vi "Interface.vi"() -> ()   [LabVIEW 2016, in "Socket Auto Connect.lvclass"]
uses:
  Socket Auto Connect.lvclass
  Robot/Universal Robot/Universal Robot.lvclass
  C:/_Code/Development/URLabVIEWInterface/Classes/Application/Application Interfaces/Application Interface/Application Interface.lvclass
  Socket Auto Connect.lvclass/Socket Auto Connect.ctl
  Client Interfaces/Socket Communication/Socket Communication.lvclass
  Application.lvclass
  Application Interface/Application Interface.lvclass
panel:
  out "connected":bool
  out "running":bool
  out "Data Viewer":string
  in  "interface":refnum<class "Socket Auto Connect.lvclass">
  in  "robot":refnum<class "Universal Robot.lvclass">
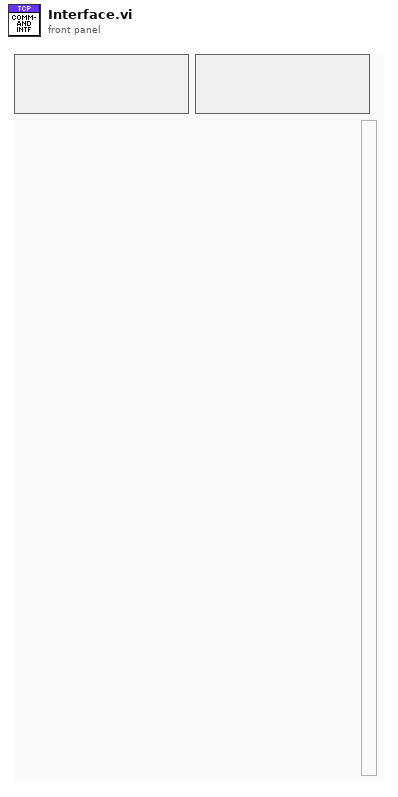
[diagram p1: front panel]
types:
  T1 = typedef "Application.lvclass/FrontPanelControls.ctl" = cluster{"Operation Interface":refnum<vi>, "Program Interface":refnum<vi>, "Command Interface":refnum<vi>, "Socket Interface":refnum<vi>}
  T2 = typedef "Universal Robot.lvclass/ProgramStatus.ctl" = cluster{"Loaded Program":string, "Valid Program":bool, "Program State":T3, "Running":bool}
  T3 = typedef "Universal Robot.lvclass/ProgramState.ctl" = enum16{"STOPPED", "PLAYING", "PAUSE"}
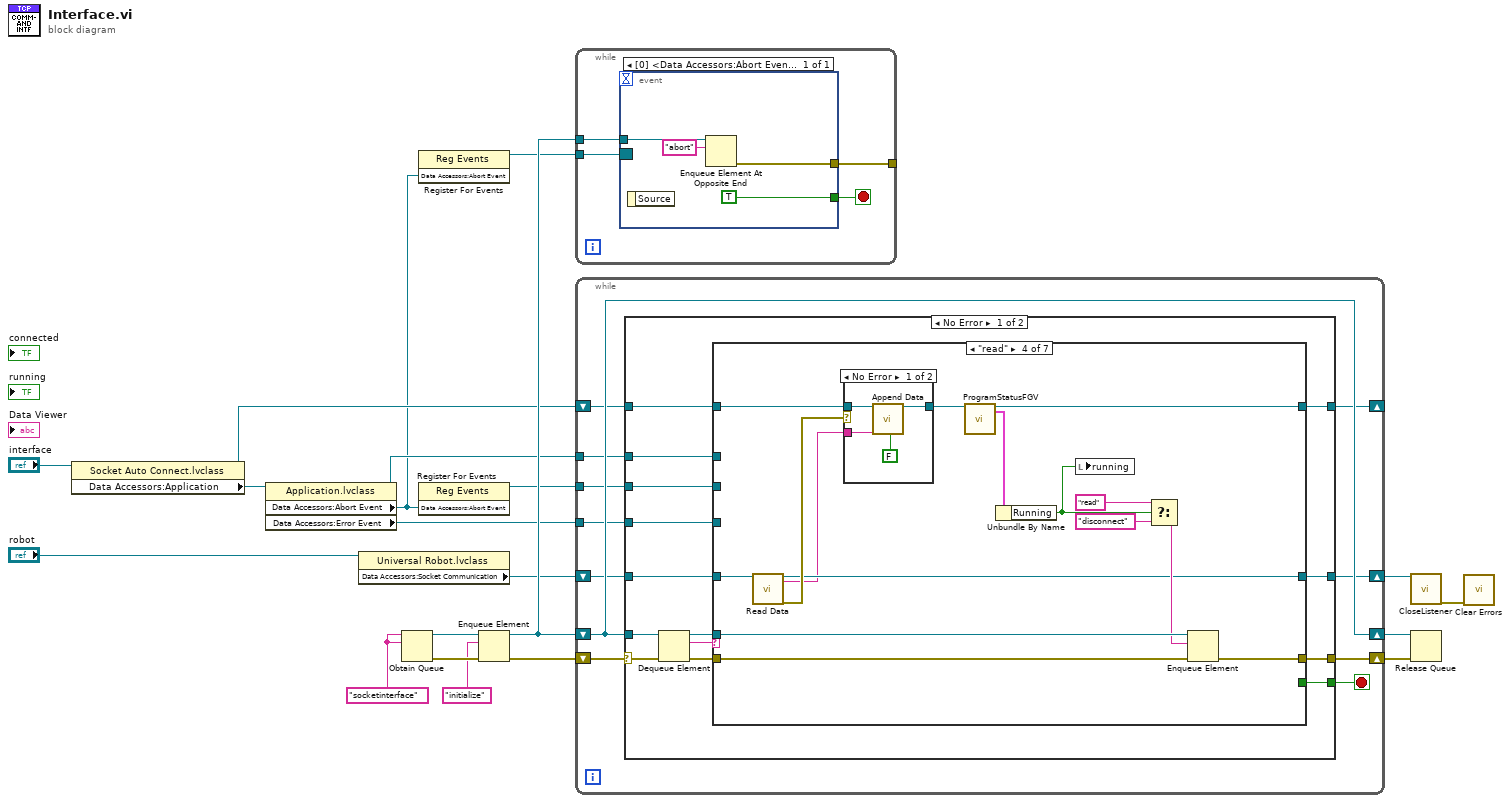
[diagram p0: block diagram]
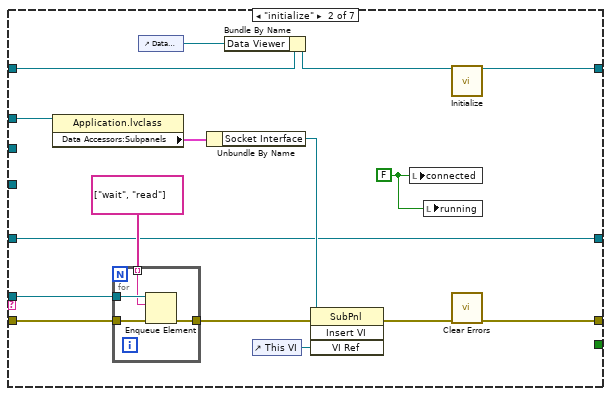
[diagram p3: hidden frame]
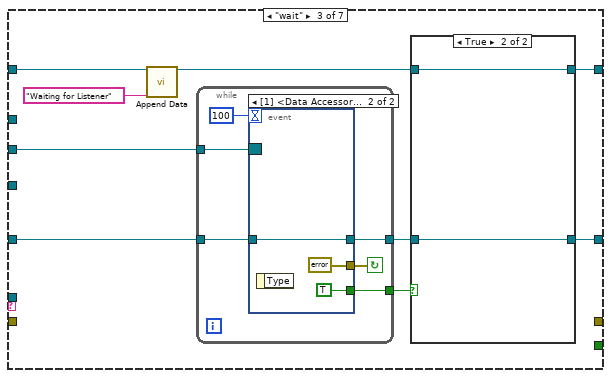
[diagram p4: hidden frame]
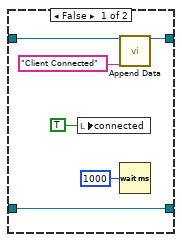
[diagram p5: hidden frame]
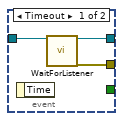
[diagram p6: hidden frame]
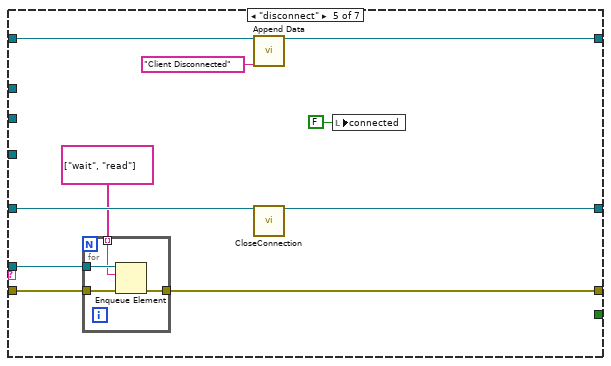
[diagram p8: hidden frame]
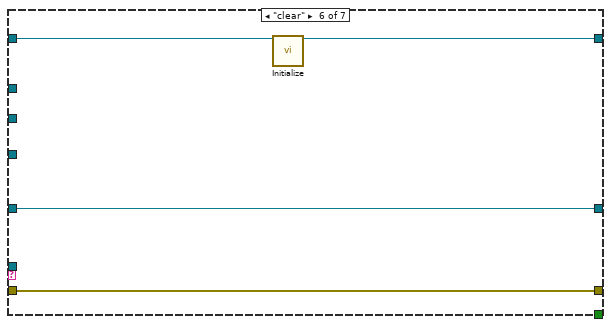
[diagram p9: hidden frame]
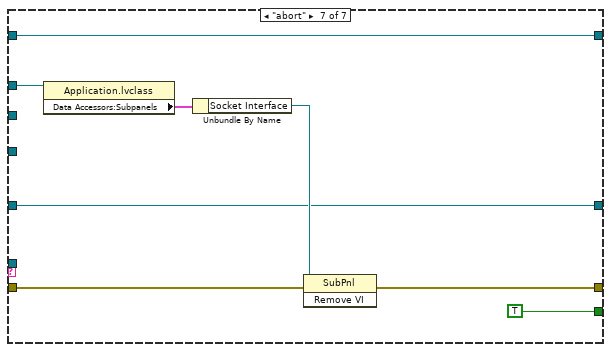
[diagram p10: hidden frame]
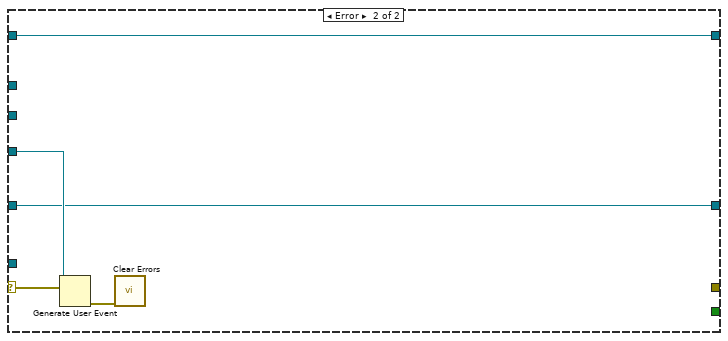
[diagram p11: hidden frame]
diagram:
  w15 = "socketinterface" ("name (unnamed)")
  n1 = property class="Socket Auto Connect.lvclass"(reference="interface") -> (reference out=w9:refnum<class "Socket Auto Connect.lvclass">, "Data Accessors:Application"=w12:refnum<class "Application.lvclass">)  [unwired: 1 in, 1 out]
  n2 = property class="Application.lvclass"(reference=w12) -> (reference out=w8:refnum<class "Application.lvclass">, "Data Accessors:Abort Event"=w3:refnum<user-event>, "Data Accessors:Error Event"=w11:refnum<user-event>)  [unwired: 1 in, 1 out]
  n3 = property class="Universal Robot.lvclass"(reference="robot") -> ("Data Accessors:Socket Communication"=w6:refnum<class "Socket Communication.lvclass">)  [unwired: 1 in, 2 out]
  n4 = Obtain Queue(name (unnamed)=w15, element data type=w15) -> (queue out=w19:refnum<queue>, error out=w20:errorcluster)  [unwired: 3 in, 1 out]
  n5 = register-events(w3) -> (reference out=w4:refnum<event-registration>)  [unwired: 2 in, 1 out]
  n6 = register-events(w3) -> (reference out=w5:refnum<event-registration>)  [unwired: 2 in, 1 out]
  n7 = Enqueue Element(queue=w19, element="initialize", error in (no error)=w20) -> (queue out=w16:refnum<queue>, error out=w17:errorcluster)  [unwired: 1 in, 1 out]
  n8 = while {
    tunnel: w16 -> [w24]
    tunnel: w4 -> [w23]
    tunnel: [w22] -> _
    stop <- w21 stop-if-true
    n9 = event shown="[0] <Data Accessors:Abort Event>: User Event" {
      selector: w23 -> [_]
      dyn-events: _ -> [_]
      timeout: _ -> [_]
      tunnel: w24 -> [w28]
      tunnel: [w27] -> w22
      tunnel: [TRUE] -> w21
      event User Event {
        n10 = event-data() -> ()  [unwired: 1 in, 1 out]
        n11 = Enqueue Element At Opposite End(queue=w28, element="abort") -> (error out=w27:errorcluster)  [unwired: 2 in, 2 out]
      }
    }
  }
  n12 = while {
    shift-right: [w37] -> w13
    shift-left: w17 -> [w39]
    shift-right: [w38] -> w14
    shift-left: w16 -> [w38]
    tunnel: w11 -> [w35]
    tunnel: w5 -> [w34]
    shift-right: [w32] -> _
    shift-left: w9 -> [w33]
    tunnel: w8 -> [w31]
    shift-right: [w29] -> w2
    shift-left: w6 -> [w30]
    stop <- w36 stop-if-true
    n13 = case shown="No Error" w39 {
      selector: w39 -> [w52 w156]
      tunnel: w38 -> [w53 _]
      tunnel: [w48 _] -> w37
      tunnel: [w47 _] -> w36
      tunnel: w35 -> [w46 w154]
      tunnel: w34 -> [w45 _]
      tunnel: w33 -> [w44 w153]
      tunnel: [w43 w153] -> w32
      tunnel: w31 -> [w42 _]
      tunnel: w30 -> [w41 w152]
      tunnel: [w40 w152] -> w29
      frame No Error {
        n14 = Dequeue Element(queue=w53, error in (no error)=w52) -> (queue out=w49:refnum<queue>, element=w50:string, error out=w51:errorcluster)  [unwired: 1 in, 1 out]
        n15 = case shown="\"read\"" w50 {
          tunnel: w51 -> [w56 w63 _ w113 w127 w142 w150]
          tunnel: w49 -> [_ w64 _ w114 w128 _ _]
          tunnel: [w56 w58 _ w111 w126 w142 w149] -> w48
          tunnel: [_ _ _ _ _ _ TRUE] -> w47
          tunnel: w46 -> [_ _ _ _ _ _ _]
          tunnel: w45 -> [_ _ w85 _ _ _ _]
          tunnel: w44 -> [w55 w69 w84 w116 w135 w141 w146]
          tunnel: [w55 w67 w81 w120 w134 w140 w146] -> w43
          tunnel: w42 -> [_ w65 _ _ _ _ w145]
          tunnel: w41 -> [w54 w57 w79 w118 w131 w143 w144]
          tunnel: [w54 w57 w77 w107 w130 w143 w144] -> w40
          frame Default {
          }
          frame "initialize" {
            w60 = FALSE ("connected")
            n16 = property class="Application.lvclass"(reference=w65) -> ("Data Accessors:Subpanels"=w71:T1)  [unwired: 1 in, 2 out]
            n17 = for {
              tunnel: w64 -> [w76]
              tunnel: w63 -> [w75]
              tunnel: [w74] -> w62
              tunnel: string[] ["wait", "read"] -> [w73] mode=indexing
              n18 = Enqueue Element(queue=w76, element=w73, error in (no error)=w75) -> (error out=w74:errorcluster)  [unwired: 1 in, 2 out]
            }
            n19 = control-ref of="Data Viewer"() -> (w68:refnum<vi>)
            n20 = Unbundle By Name(w71) -> ("Socket Interface"=w70:refnum<vi>)
            n21 = Bundle By Name(cluster=w69, "Data Viewer"=w68) -> (w66:refnum<class "Socket Auto Connect.lvclass">)
            n22 = control-ref of="This VI"() -> (w72:refnum<vi>)
            n23 = invoke class="SubPnl" method="Insert VI"(reference=w70, error in=w62, "VI Ref"=w72) -> (error out=w59:errorcluster)  [unwired: 1 in, 3 out]
            n24 = local write "connected"(w60) -> ()
            n25 = local write "running"(w60) -> ()
            n26 = call "Initialize.vi"("Socket Auto Connect in"=w66) -> ("Socket Auto Connect out"=w67:refnum<class "Socket Auto Connect.lvclass">)  [unwired: 17 in, 1 out]
            n27 = call <vilib>:"Clear Errors.vi"("error in (no error)"=w59) -> ("error out"=w58:errorcluster)  [unwired: 5 in, 1 out]
          }
          frame "wait" {
            n28 = call "Append Data.vi"("Socket Auto Connect in"=w84, "String to Append"="Waiting for Listener") -> ("Socket Auto Connect out"=w82:refnum<class "Socket Auto Connect.lvclass">)  [unwired: 16 in, 1 out]
            n29 = while {
              tunnel: w79 -> [w99]
              tunnel: w85 -> [w97]
              tunnel: [w95] -> w80
              tunnel: [w94] -> w78
              stop <- w96 continue-if-true
              n30 = event shown="[1] <Data Accessors:Abort Event>: User Event" {
                selector: w97 -> [_ _]
                dyn-events: _ -> [_ _]
                timeout: 100 -> [_ _]
                tunnel: w99 -> [w102 w104]
                tunnel: [w101 errorcluster {"status"=FALSE, "code"=0, "source"=""} ("error out")] -> w96
                tunnel: [_ TRUE] -> w95
                tunnel: [w100 w104] -> w94
                event Timeout {
                  n31 = event-data() -> ()  [unwired: 1 in, 1 out]
                  n32 = call "WaitForListener.vi"("Socket Listener in"=w102) -> ("Socket Listener out"=w100:refnum<class "Socket Communication.lvclass">, "error out"=w101:errorcluster)  [unwired: 17 in]
                }
                event User Event {
                  n33 = event-data() -> ()  [unwired: 1 in, 1 out]
                }
              }
            }
            n34 = case shown="True" w80 {
              tunnel: w82 -> [w91 w93]
              tunnel: [w90 w93] -> w81
              tunnel: w78 -> [w86 w92]
              tunnel: [w86 w92] -> w77
              frame False {
                n35 = local write "connected"(TRUE ("connected")) -> ()
                n36 = call "Append Data.vi"("Socket Auto Connect in"=w91, "String to Append"="Client Connected") -> ("Socket Auto Connect out"=w90:refnum<class "Socket Auto Connect.lvclass">)  [unwired: 16 in, 1 out]
                n37 = Wait (ms)(milliseconds to wait=u32 1000) -> ()  [unwired: 1 out]
              }
              frame True {
              }
            }
          }
          frame "read" {
            n38 = call-dynamic "Read Data.vi"("TCP Socket in"=w118) -> ("TCP Socket out"=w107:refnum<class "Socket Communication.lvclass">, "data"=w106:string, "error out"=w115:errorcluster)  [unwired: 16 in]
            n39 = case shown="No Error" w115 {
              tunnel: [w124 w125] -> w117
              tunnel: w116 -> [w123 w125]
              tunnel: w106 -> [w122 _]
              frame No Error {
                n40 = call "Append Data.vi"("Socket Auto Connect in"=w123, "String to Append"=w122, "Return (T)"=FALSE) -> ("Socket Auto Connect out"=w124:refnum<class "Socket Auto Connect.lvclass">)  [unwired: 15 in, 1 out]
              }
              frame Error {
              }
            }
            n41 = call "ProgramStatusFGV.vi"("Application Interface in"=w117) -> ("Application Interface out"=w120:refnum<class "Socket Auto Connect.lvclass">, "Program Status out"=w119:T2)  [unwired: 16 in, 1 out]
            n42 = Unbundle By Name(w119) -> ("Running"=w108:bool)
            n43 = local write "running"(w108) -> ()
            n44 = Select(t="read", s=w108, f="disconnect") -> (s? t:f=w110:string)
            n45 = Enqueue Element(queue=w114, element=w110, error in (no error)=w113) -> (error out=w111:errorcluster)  [unwired: 1 in, 2 out]
          }
          frame "disconnect" {
            n46 = for {
              tunnel: w128 -> [w139]
              tunnel: w127 -> [w138]
              tunnel: [w137] -> w126
              tunnel: string[] ["wait", "read"] -> [w136] mode=indexing
              n47 = Enqueue Element(queue=w139, element=w136, error in (no error)=w138) -> (error out=w137:errorcluster)  [unwired: 1 in, 2 out]
            }
            n48 = call "Append Data.vi"("Socket Auto Connect in"=w135, "String to Append"="Client Disconnected") -> ("Socket Auto Connect out"=w134:refnum<class "Socket Auto Connect.lvclass">)  [unwired: 16 in, 1 out]
            n49 = call-dynamic "CloseConnection.vi"("TCP Socket in"=w131) -> ("TCP Socket out"=w130:refnum<class "Socket Communication.lvclass">)  [unwired: 17 in, 1 out]
            n50 = local write "connected"(FALSE ("connected")) -> ()
          }
          frame "clear" {
            n51 = call "Initialize.vi"("Socket Auto Connect in"=w141) -> ("Socket Auto Connect out"=w140:refnum<class "Socket Auto Connect.lvclass">)  [unwired: 17 in, 1 out]
          }
          frame "abort" {
            n52 = property class="Application.lvclass"(reference=w145) -> ("Data Accessors:Subpanels"=w148:T1)  [unwired: 1 in, 2 out]
            n53 = Unbundle By Name(w148) -> ("Socket Interface"=w147:refnum<vi>)
            n54 = invoke class="SubPnl" method="Remove VI"(reference=w147, error in=w150) -> (error out=w149:errorcluster)  [unwired: 1 in, 2 out]
          }
        }
      }
      frame Error {
        n55 = Generate User Event(user event=w154, event data cluster=w156) -> (error out=w155:errorcluster)  [unwired: 2 in, 1 out]
        n56 = call <vilib>:"Clear Errors.vi"("error in (no error)"=w155) -> ()  [unwired: 5 in, 2 out]
      }
    }
  }
  n57 = call-dynamic "CloseListener.vi"("TCP Socket in"=w2) -> ("error out"=w1:errorcluster)  [unwired: 17 in, 1 out]
  n58 = Release Queue(queue=w14, error in (no error)=w13) -> ()  [unwired: 1 in, 3 out]
  n59 = call <vilib>:"Clear Errors.vi"("error in (no error)"=w1) -> ()  [unwired: 5 in, 2 out]
